vi "Autonomous Independent.vi"   [LabVIEW 2016]
doc: "This VI is called when autonomous begins, and will automatically be terminated when autonomous ends. You can carry out timed or sensor driven robot movement independently without needing to return to the caller."
uses:
  <vilib>/Rock Robotics/Network Tables/NT Read String.vi
  Robot Global Data.vi
panel:
  # "Be sure to right-click and choose Data Operations>>Make Current Value default if you want to save the array values with the VI"
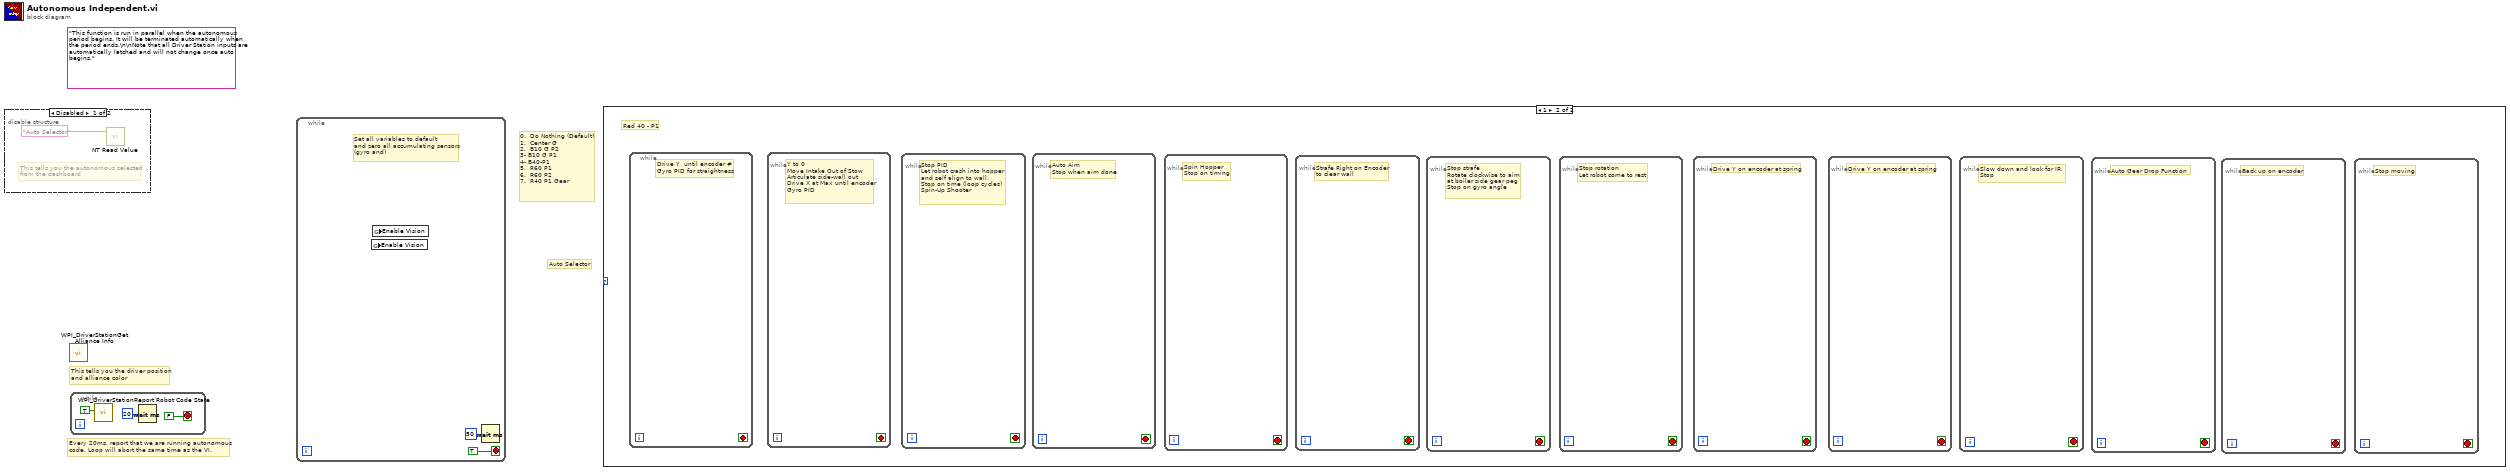
[diagram p0: block diagram]
diagram:
  (unwired) "This function is run in parallel when the autonomous period begins. It will be terminated automatically when the period ends.\n\nNote that all Driver Station inputs are automatically latched and will not change once auto begins."
  # "0.  Do Nothing (Default)\n1.  Center G\n2.  B10 G P2\n3- B10 G P1\n4- B40-P1\n5.  R60 P1\n6.  R60 P2\n7.  R40 P1 Gear"
  # "Auto Selector"
  # "Every 20ms, report that we are running autonomous\ncode. Loop will abort the same time as the VI."
  # "This tells you the driver position\nand alliance color"
  n1 = disable-structure shown="Disabled" {
    frame Disabled {
      # "This tells you the autonomous selected\nfrom the dashboard"
      n2 = call-poly <vilib>:"NT Read Value.vi"("Name"="Auto Selector") -> ()  [unwired: 9 in, 2 out]
    }
    frame Enabled {
    }
  }
  n3 = call <vilib>:"WPI_DriverStationGet Alliance Info.vi"() -> ()  [unwired: 12 out]
  n4 = while {
    stop <- FALSE stop-if-true
    n5 = call <vilib>:"WPI_DriverStationReport Robot Code State.vi"("Autonomous"=TRUE) -> ()  [unwired: 10 in, 1 out]
    n6 = Wait (ms)(milliseconds to wait=u32 20) -> ()  [unwired: 1 out]
  }
  n7 = while {
    stop <- TRUE stop-if-true
    # "Set all variables to default\nand zero all accumulating sensors\n(gyro and)"
    n8 = global read "Robot Global Data.vi" "Enable Vision"() -> ()  [unwired: 1 in]
    n9 = global read "Robot Global Data.vi" "Enable Vision"() -> ()  [unwired: 1 in]
    n10 = Wait (ms)(milliseconds to wait=u32 50) -> ()  [unwired: 1 out]
  }
  n11 = case shown="1" {
    selector: _ -> [_ _]
    frame 0, Default {
    }
    frame 1 {
      # "Red 40 - P1"
      n12 = while {
        stop <- _ stop-if-true
        # "Drive Y  until encoder #\nGyro PID for straightness"
      }
      n13 = while {
        stop <- _ stop-if-true
        # "Y to 0\nMove Intake Out of Stow\nArticulate side-wall out\nDrive X at Max until encoder\nGyro PID"
      }
      n14 = while {
        stop <- _ stop-if-true
        # "Stop PID\nLet robot crash into hopper\nand self align to wall.\nStop on time (loop cycles)\nSpin-Up Shooter"
      }
      n15 = while {
        stop <- _ stop-if-true
        # "Auto Aim\nStop when aim done"
      }
      n16 = while {
        stop <- _ stop-if-true
        # "Spin Hopper\nStop on timing"
      }
      n17 = while {
        stop <- _ stop-if-true
        # "Strafe Right on Encoder\nto clear wall"
      }
      n18 = while {
        stop <- _ stop-if-true
        # "Stop strafe\nRotate clockwise to aim\nat boiler side gear peg\nStop on gyro angle"
      }
      n19 = while {
        stop <- _ stop-if-true
        # "Stop rotation\nLet robot come to rest"
      }
      n20 = while {
        stop <- _ stop-if-true
        # "Drive Y on encoder at spring"
      }
      n21 = while {
        stop <- _ stop-if-true
        # "Drive Y on encoder at spring"
      }
      n22 = while {
        stop <- _ stop-if-true
        # "Slow down and look for IR.  \nStop"
      }
      n23 = while {
        stop <- _ stop-if-true
        # "Auto Gear Drop Function"
      }
      n24 = while {
        stop <- _ stop-if-true
        # "Back up on encoder"
      }
      n25 = while {
        stop <- _ stop-if-true
        # "Stop moving"
      }
    }
  }
